vi "EvaluateShot.vi"(5 "Gap Coord":dbl[](array[numeric]), 7 "BestY":dbl, 8 "error in (no error)":errorcluster, 9 "Game":refnum<class "Game.lvclass">, 10 "Point":dbl[](array[numeric]), 11 "object in":refnum<class "Utilities.lvclass">) -> (0 "error out":errorcluster, 2 "Evaluation":dbl, 3 "object out":refnum<class "Utilities.lvclass">)   [LabVIEW 2023, in "Utilities.lvclass"]
uses:
  Utilities.lvclass
  Game_class/Game.lvclass
  Game_class/Game.lvclass/Game.ctl
  Parameters_class/Parameters.lvclass/Parameters.ctl
  Game_class/Read Parameters.lvclass.vi
  Parameters_class/Read AttakingOurselves.vi
  Parameters_class/Parameters.lvclass
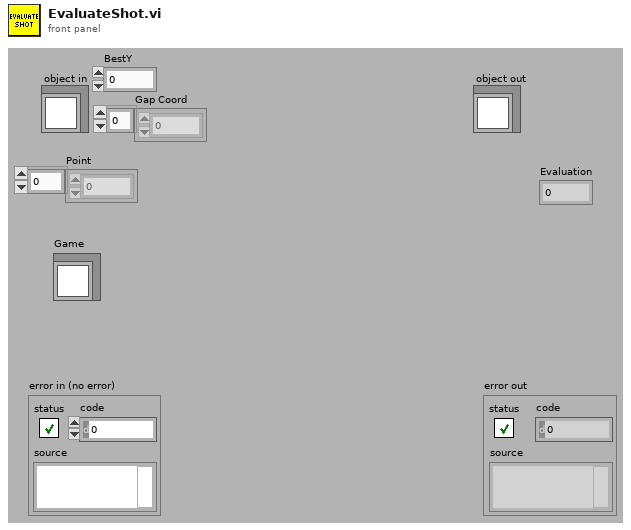
[diagram p1: front panel]
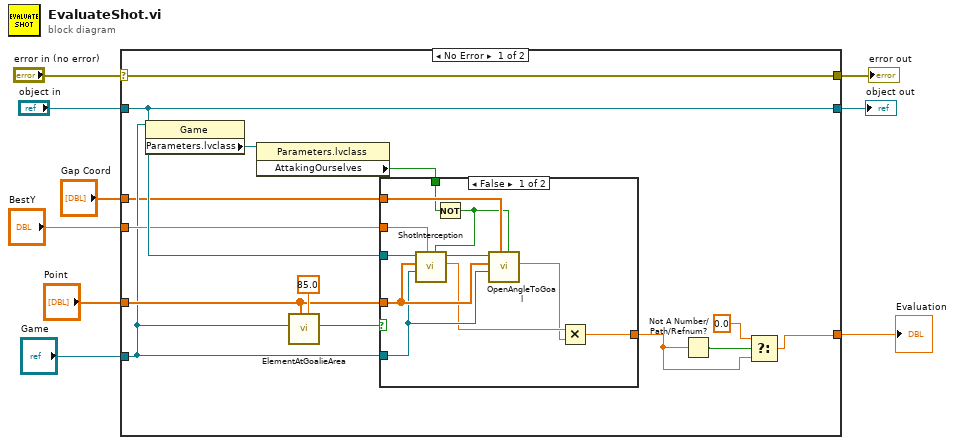
[diagram p0: block diagram]
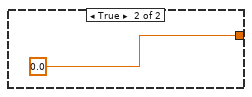
[diagram p2: hidden frame]
diagram:
  n1 = case shown="No Error" "error in (no error)" {
    selector: "error in (no error)" -> [w23 w37]
    tunnel: [w23 w37] -> w8
    tunnel: [w21 w36] -> w6
    tunnel: "object in" -> [w21 w36]
    tunnel: "Point" -> [w20 _]
    tunnel: "Game" -> [w18 _]
    tunnel: [w12 _] -> w3
    tunnel: "BestY" -> [w19 _]
    tunnel: "Gap Coord" -> [w15 _]
    frame No Error {
      n2 = property class="Game"(reference=w18) -> ("Parameters.lvclass"=w17:refnum<class "Parameters.lvclass">)  [unwired: 1 in, 2 out]
      n3 = property class="Parameters.lvclass"(reference=w17) -> ("AttakingOurselves"=w16:bool)  [unwired: 1 in, 2 out]
      n4 = call "ElementAtGoalieArea.vi"("ElementRadius"=85.0, "Elemento pos."=w20, "Game"=w18) -> ("Element at any goalkeeper area ?"=w14:bool)  [unwired: 4 in, 4 out]
      n5 = case shown="False" w14 {
        tunnel: [w29 0.0 ("ElementRadius")] -> w11
        tunnel: w21 -> [w34 _]
        tunnel: w20 -> [w31 _]
        tunnel: w19 -> [w33 _]
        tunnel: w18 -> [w30 _]
        tunnel: w16 -> [w27 _]
        tunnel: w15 -> [w28 _]
        frame False {
          n6 = Not(x=w27) -> (.not. x?=w25:bool)
          n7 = call-dynamic "ShotInterception.vi"("Ally?"=w25, "BestY"=w33, "Game"=w30, "Point"=w31, "object in"=w34) -> ("Evaluation"=w26:dbl, "object out"=w32:refnum<class "Utilities.lvclass">)  [unwired: 4 in, 1 out]
          n8 = call "OpenAngleToGoal.vi"("Ally?"=w25, "Gap Coord"=w28, "Game"=w30, "Point"=w31, "object in"=w32) -> ("Evaluation"=w24:dbl)  [unwired: 4 in, 2 out]
          n9 = Multiply(x=w26, y=w24) -> (x*y=w29:dbl)
        }
        frame True {
        }
      }
      n10 = Not A Number/Path/Refnum?(number/path/refnum=w11) -> (NaN/Path/Refnum?=w10:bool)
      n11 = Select(t=0.0, s=w10, f=w11) -> (s? t:f=w12:dbl)
    }
    frame Error {
    }
  }
  "error out" <- w8
  "object out" <- w6
  "Evaluation" <- w3
